vi "DecodeVSSRef_Command.vi"(1 "element":u8[](array[numeric]), 5 "error in (no error)":errorcluster) -> (17 "VSS_Ref 3":T1={"FoulQuadrantVSS"=enum."NO_QUADRANT", "TeamColorVSS"=enum."YELLOW", "HalfVSS"=enum."NO_HALF", "Foul"=enum."FREE_KICK", "timestamp"=0.0}, 19 "error out":errorcluster)   [LabVIEW 2023, in "Referee.lvclass"]
uses:
  Referee.lvclass
  Control 6.ctl
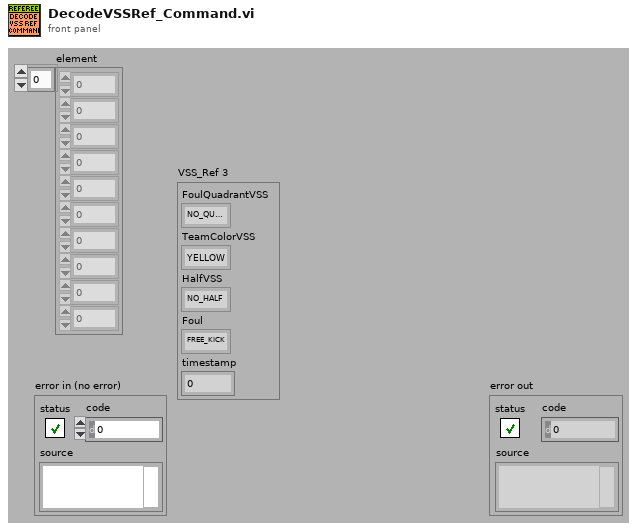
[diagram p1: front panel]
types:
  T1 = typedef "Control 6.ctl" = cluster{"FoulQuadrantVSS":enum16{"NO_QUADRANT", "QUADRANT_1", "QUADRANT_2", "QUADRANT_3", "QUADRANT_4"}, "TeamColorVSS":enum16{"BLUE", "YELLOW", "NONE"}, "HalfVSS":enum16{"NO_HALF", "FIRST_HALF", "SECOND_HALF", "OVERTIME_FIRST_HALF", "OVERTIME_SECOND_HALF", "PENALTY_SHOOTOUS"}, "Foul":enum16{"FREE_KICK", "PENALTY_KICK", "GOAL_KICK", "FREE_BALL", "KICKOFF", "STOP", "GAME_ON", "HALT"}, "timestamp":dbl}
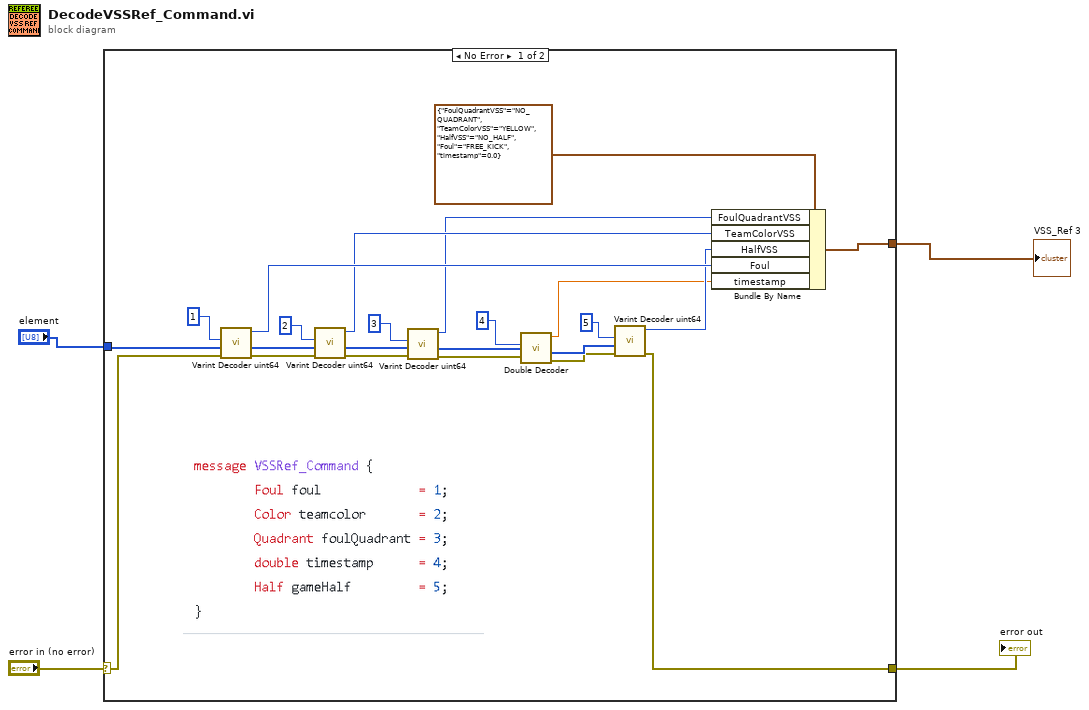
[diagram p0: block diagram]
diagram:
  n1 = case shown="No Error" "error in (no error)" {
    selector: "error in (no error)" -> [w11 w28]
    tunnel: [w6 w28] -> w3
    tunnel: "element" -> [w24 _]
    tunnel: [w26 _] -> w1
    frame No Error {
      n2 = call "Varint Decoder uint64.vi"("error in (no error)"=w11, "Array"=w24, "Key"=1) -> ("error out"=w10:errorcluster, "array w/ subset deleted"=w22:u8[], "Varint"=w23:u64)  [unwired: 5 in, 1 out]
      n3 = call "Varint Decoder uint64.vi"("error in (no error)"=w10, "Array"=w22, "Key"=2) -> ("error out"=w9:errorcluster, "array w/ subset deleted"=w18:u8[], "Varint"=w20:u64)  [unwired: 5 in, 1 out]
      n4 = call "Varint Decoder uint64.vi"("error in (no error)"=w9, "Array"=w18, "Key"=3) -> ("error out"=w8:errorcluster, "array w/ subset deleted"=w17:u8[], "Varint"=w16:u64)  [unwired: 5 in, 1 out]
      n5 = call "Double Decoder.vi"("error in (no error)"=w8, "Array"=w17, "Key"=4) -> ("error out"=w7:errorcluster, "array w/ subset deleted"=w14:u8[], "Double"=w12:dbl)  [unwired: 5 in, 1 out]
      n6 = call "Varint Decoder uint64.vi"("error in (no error)"=w7, "Array"=w14, "Key"=5) -> ("error out"=w6:errorcluster, "Varint"=w15:u64)  [unwired: 5 in, 2 out]
      n7 = Bundle By Name(cluster=T1 {"FoulQuadrantVSS"=enum."NO_QUADRANT", "TeamColorVSS"=enum."YELLOW", "HalfVSS"=enum."NO_HALF", "Foul"=enum."FREE_KICK", "timestamp"=0.0} ("VSS_Ref 2"), "FoulQuadrantVSS"=w16, "TeamColorVSS"=w20, "HalfVSS"=w15, "Foul"=w23, "timestamp"=w12) -> (w26:T1)
    }
    frame Error {
    }
  }
  "error out" <- w3
  "VSS_Ref 3" <- w1
